vi "CSM - Set Module Attribute.vi"(0 "CSM Name":string, 5 "Attribute":string, 7 "Value":variant, 9 "Wait (5000 ms)":i32=5000, 11 "Error In":errorcluster caption="error in (no error)") -> (4 "CSM Name (Dup)":string, 6 "Replaced":bool, 10 "Waited (ms)":u32, 15 "error out":errorcluster)   [LabVIEW 2017, in "Communicable State Machine.lvlib"]
doc: "Sets the attribute value of the specified module. If the attribute does not exist, a new attribute is created, and <b>Replaced</b> returns FALSE. Otherwise, it returns TRUE. If the CSM module does not exist, this VI waits for the specified timeout duration. If the timeout is exceeded, this VI returns a timeout error.\n\n\n> [!NOTE] <b>CSM Module Attributes</b>\n>\n> CSM module attributes are a data area that can store module configuration and status, accessed by name. CSM module attributes can be used in the following scenarios:\n> - Providing a way to access and modify configuration and status information without messages. For example, a \"Connected\" attribute in a TCP module indicating whether a connection is established is more convenient to access directly.\n> - Nodes running in advanced modes, such as Worker Mode and Chain of Responsibility Mode, share the same data area, which is used for sharing data between modules.\n\n\n<b>Reference Example</b>: `[CSM-Example]\\0. Base Concepts\\6. Module Attributes.vi`.\n\n-- <b>Controls</b> --\n- <b>CSM Name</b>: CSM module name.\n- <b>Attribute</b>: Attribute name. Must not be an empty string.\n- <b>Value</b>: Attribute data.\n- <b>Wait (5000 ms)</b>: Timeout duration for waiting module to be alive. The default is 5000 ms.\n\n-- <b>Indicators</b> --\n- <b>CSM Name (Dup)</b>: A copy of the input CSM module name.\n- <b>Replaced</b>: Whether the attribute was replaced.\n- <b>Waited (ms)</b>: Time elapsed while waiting."
uses:
  Communicable State Machine.lvlib
  _Support/CSMQ/_CSMOFGV(lvlibp).vi
  CSM - Wait for Module to Be Alive.vi
  _Shared/CSM Shared.lvlib
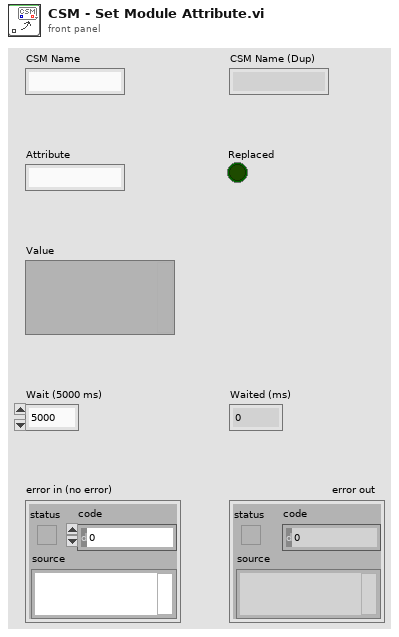
[diagram p1: front panel]
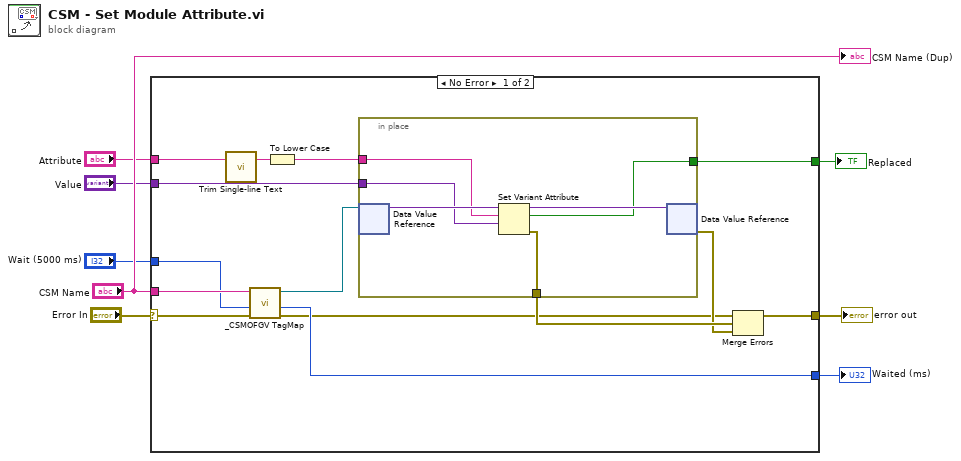
[diagram p0: block diagram]
diagram:
  n1 = case shown="No Error" "Error In" {
    selector: "Error In" -> [w15 w29]
    tunnel: [w22 w29] -> w7
    tunnel: "CSM Name" -> [w16 _]
    tunnel: "Attribute" -> [w21 _]
    tunnel: "Value" -> [w20 _]
    tunnel: [w17 _] -> w3
    tunnel: [w14 _] -> w2
    tunnel: "Wait (5000 ms)" -> [w13 _]
    frame No Error {
      n2 = call "Trim Single-line Text.vi"("single-line text"=w21) -> ("trimed text"=w10:string)  [unwired: 2 in]
      n3 = call "_CSMOFGV TagMap.vi"("error in (no error)"=w15, "Wait (5000 ms)"=w13, "CSM Name"=w16) -> ("error out"=w12:errorcluster, "Waited (ms)"=w14:u32, "TagMap"=w11:refnum<data-value>)  [unwired: 6 in]
      n4 = To Lower Case(string=w10) -> (all lower case string=w9:string)
      n5 = in-place {
        in-place-border: w9 -> [w26]
        in-place-border: w20 -> [w25]
        in-place-border: [w24] -> w19
        in-place-border: [w23] -> w17
        n6 = in-place-dvr #1(w11) -> (w28:variant)  [unwired: 1 out]
        n7 = Set Variant Attribute(Variant=w28, name=w26, value=w25) -> (Variant out=w27:variant, replaced=w23:bool, error out=w24:errorcluster)  [unwired: 1 in]
        n8 = in-place-dvr #1(w27) -> (w18:errorcluster)  [unwired: 1 out]
      }
      n9 = Merge Errors(w12, w19, w18) -> (w22:errorcluster)
    }
    frame Error {
    }
  }
  "error out" <- w7
  "Replaced" <- w3
  "Waited (ms)" <- w2
  "CSM Name (Dup)" <- "CSM Name"
